vi "Set ComboCell DataSource (String).vi"(0 "DataGridView in":refnum<class "DataGridView.lvclass">, 5 "row index":i32, 7 "col index":i32, 9 "Combo DataSource":string[](array[string]), 11 "error in":errorcluster) -> (4 "DataGridView out":refnum<class "DataGridView.lvclass">, 15 "error out":errorcluster)   [LabVIEW 2016, in "DataGrid.lvlib" / "DataGridView.lvclass"]
uses:
  <userlib>/LabVIEWdotNetDataGrid/source/DataGridView/DataGridView.lvclass
  System.Windows.Forms
  <userlib>/LabVIEWdotNetDataGrid/source/DataGridView/DataGridView.lvclass/DataGridView.ctl
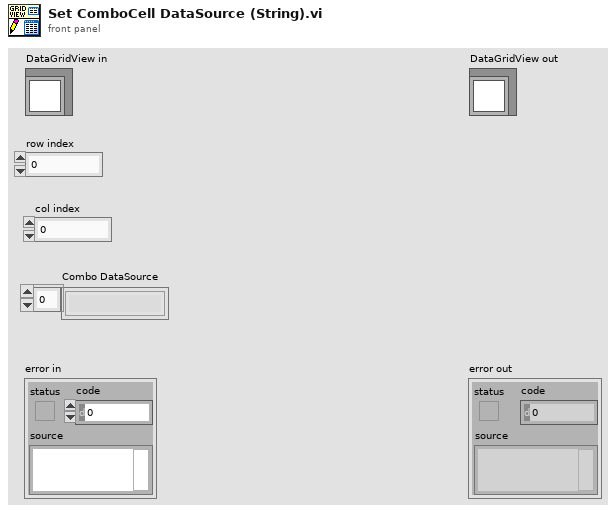
[diagram p1: front panel]
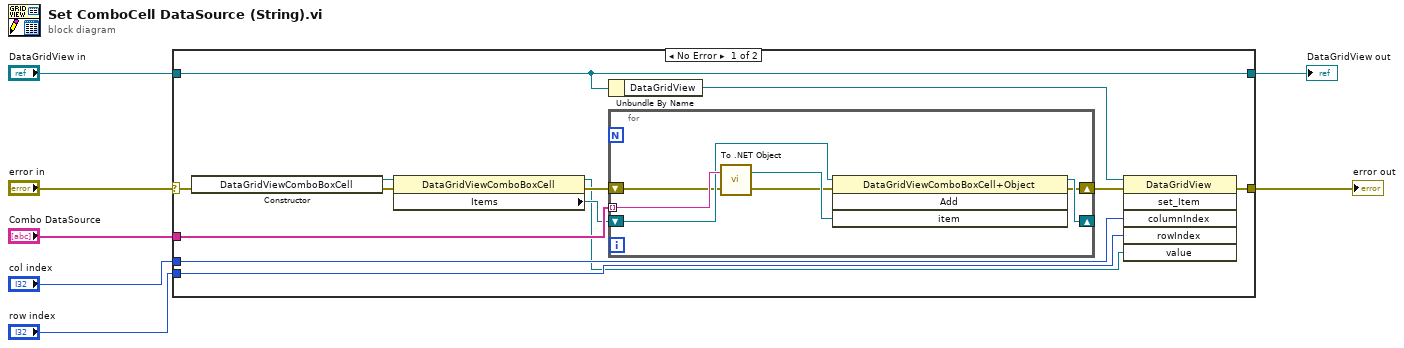
[diagram p0: block diagram]
diagram:
  n1 = case shown="No Error" "error in" {
    selector: "error in" -> [w11 w28]
    tunnel: [w8 w28] -> w6
    tunnel: [w20 w29] -> w4
    tunnel: "DataGridView in" -> [w20 w29]
    tunnel: "Combo DataSource" -> [w16 _]
    tunnel: "col index" -> [w18 _]
    tunnel: "row index" -> [w17 _]
    frame No Error {
      n2 = constructor class="DataGridViewComboBoxCell"(error in=w11) -> (reference out=w13:refnum<k24>, error out=w12:errorcluster)  [unwired: 2 in, 1 out]
      n3 = property class="DataGridViewComboBoxCell"(reference=w13, error in=w12) -> (reference out=w10:refnum<k24>, error out=w14:errorcluster, "Items"=w15:refnum<k24>)
      n4 = Unbundle By Name(w20) -> ("DataGridView"=w19:refnum<k24>)
      n5 = for {
        tunnel: w16 -> [w27] mode=indexing
        shift-right: [w24] -> _
        shift-left: w15 -> [w26]
        shift-right: [w21] -> w9
        shift-left: w14 -> [w23]
        n6 = call <vilib>:"To .NET Object.vi"("error in (no error)"=w23, "anything"=w27) -> ("error out"=w22:errorcluster, ".NET object"=w25:refnum<k24>)
        n7 = invoke class="DataGridViewComboBoxCell+Object" method="Add"(reference=w26, error in=w22, "item"=w25) -> (reference out=w24:refnum<k24>, error out=w21:errorcluster)  [unwired: 1 in, 2 out]
      }
      n8 = invoke class="DataGridView" method="set_Item"(reference=w19, error in=w9, "columnIndex"=w18, "rowIndex"=w17, "value"=w10) -> (error out=w8:errorcluster)  [unwired: 1 in, 5 out]
    }
    frame Error {
    }
  }
  "error out" <- w6
  "DataGridView out" <- w4
